vi "GetAgregateAlarm.vi"(0 "reference in":refnum<class "Sig_Digital.lvclass">, 11 "error in (no error)":errorcluster) -> (4 "reference out":refnum<class "Sig_Digital.lvclass">, 6 "Alarm":bool, 15 "error out":errorcluster)   [LabVIEW 2019, in "Sig_Digital.lvclass"]
uses:
  Sig_Digital.lvclass
  Sig_Digital.lvclass/Sig_Digital.ctl
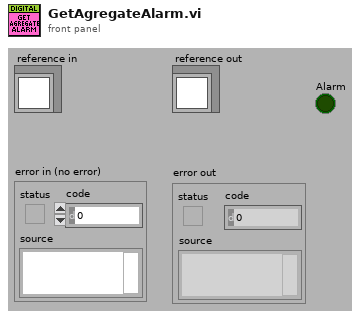
[diagram p1: front panel]
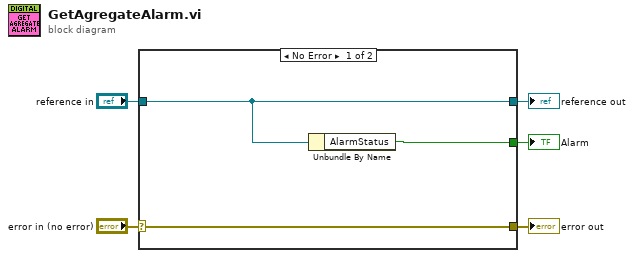
[diagram p0: block diagram]
diagram:
  n1 = case shown="No Error" "error in (no error)" {
    selector: "error in (no error)" -> [w8 w10]
    tunnel: [w8 w10] -> w4
    tunnel: [w6 w9] -> w2
    tunnel: "reference in" -> [w6 w9]
    tunnel: [w7 _] -> w1
    frame No Error {
      n2 = Unbundle By Name(w6) -> ("AlarmStatus"=w7:bool)
    }
    frame Error {
    }
  }
  "error out" <- w4
  "reference out" <- w2
  "Alarm" <- w1
